vi "Remote Panels Handler.vi"(8 "error in (no error)":errorcluster, 10 "Limit  connections":i32=1 min=1, 11 "VI in":refnum<vi>) -> (0 "error out":errorcluster, 3 "VI out":refnum<vi>)   [LabVIEW 2018]
uses:
  Remote Panels Globals.vi
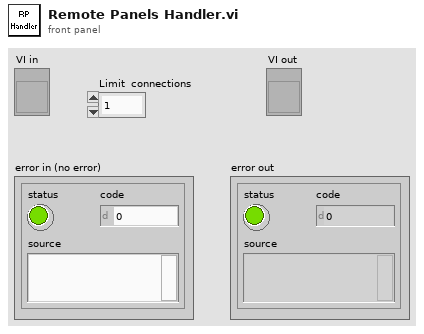
[diagram p1: front panel]
types:
  T1 = enum32{"Bad", "Idle", "Run top level", "Running"}
  T2 = typedef "LVRemotePanelConnectionsTypeDef.ctl" = cluster{"VI Name":string, "Remote":string, "UserName":string, "Port":i32, "Status":enum32{"Viewing", "Waiting For Control", "Controlling"}, "Create Time":timestamp, "Status Time":timestamp, "Control End Time":timestamp}[]
  T3 = cluster{"VI Name":string, "Remote":string, "UserName":string, "Port":i32, "Status":enum32{"Viewing", "Waiting For Control", "Controlling"}, "Create Time":timestamp, "Status Time":timestamp, "Control End Time":timestamp}
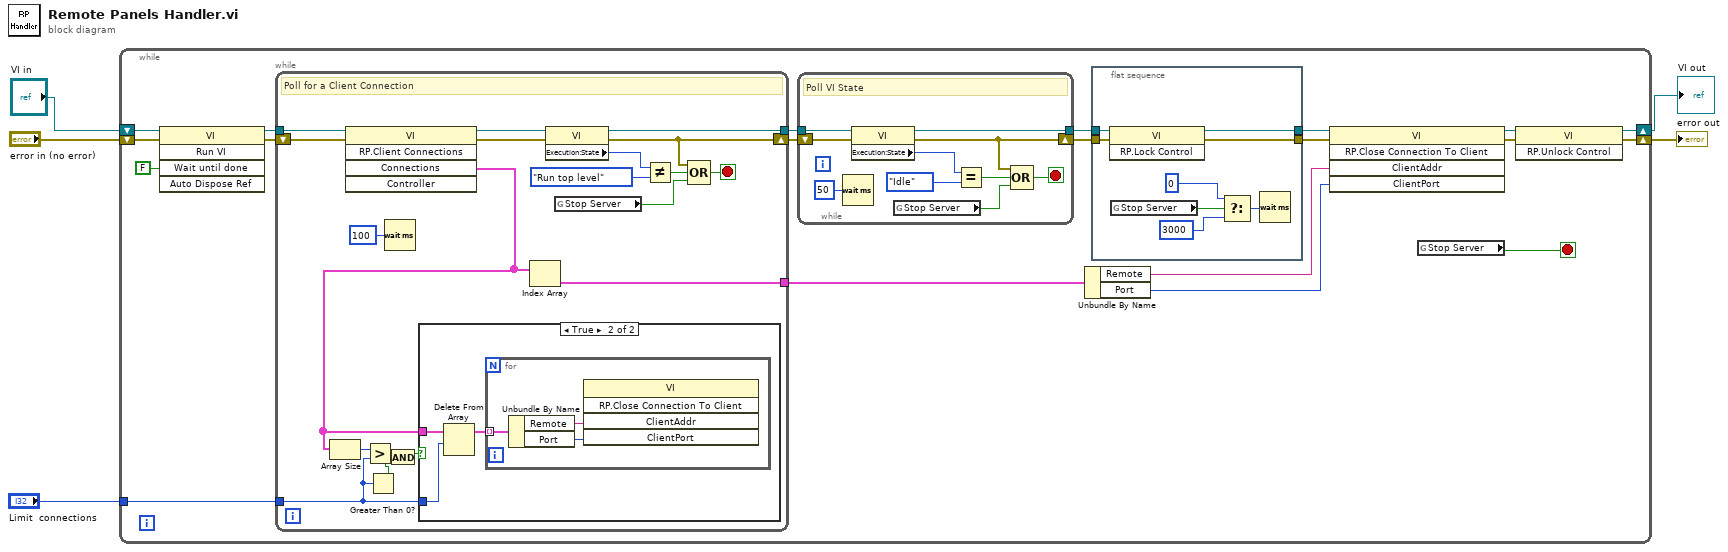
[diagram p0: block diagram]
diagram:
  n1 = while {
    shift-right: [w22] -> w3
    shift-left: "error in (no error)" -> [w8]
    shift-right: [w23] -> w2
    shift-left: "VI in" -> [w10]
    tunnel: "Limit  connections" -> [w6]
    stop <- w12 stop-if-true
    n2 = invoke class="VI" method="Run VI"(reference=w10, error in=w8, "Wait until done"=FALSE ("Wait Until Done")) -> (reference out=w9:refnum<vi>, error out=w7:errorcluster)  [unwired: 2 in, 3 out]
    n3 = while {
      tunnel: w9 -> [w51]
      tunnel: [w54] -> w20
      shift-right: [w53] -> w21
      shift-left: w7 -> [w60]
      tunnel: [w52] -> w13
      tunnel: w6 -> [w46]
      stop <- w61 stop-if-true
      # "Poll for a Client Connection"
      n4 = invoke class="VI" method="RP.Client Connections"(reference=w51, error in=w60) -> (reference out=w55:refnum<vi>, error out=w57:errorcluster, "Connections"=w47:T2)  [unwired: 3 in, 2 out]
      n5 = Array Size(array=w47) -> (size(s)=w48:i32)
      n6 = Greater?(x=w48, y=w46) -> (0:w49:bool)
      n7 = Greater Than 0?(x=w46) -> (x > 0?=w44:bool)
      n8 = Wait (ms)(milliseconds to wait=u32 100) -> ()  [unwired: 1 out]
      n9 = And(x=w49, y=w44) -> (x .and. y?=w45:bool)
      n10 = case shown="True" w45 {
        tunnel: w47 -> [_ w65]
        tunnel: w46 -> [_ w63]
        frame False {
        }
        frame True {
          n11 = Delete From Array(array=w65, length=w63) -> (array with subset deleted=w64:T2)  [unwired: 1 in, 1 out]
          n12 = for {
            tunnel: w64 -> [w68] mode=indexing
            n13 = Unbundle By Name(w68) -> ("Remote"=w67:string, "Port"=w66:i32)
            n14 = invoke class="VI" method="RP.Close Connection To Client"("ClientAddr"=w67, "ClientPort"=w66) -> ()  [unwired: 3 in, 5 out]
          }
        }
      }
      n15 = Index Array(array=w47) -> (element=w52:T3)  [unwired: 1 in]
      n16 = property class="VI"(reference=w55, error in=w57) -> (reference out=w54:refnum<vi>, error out=w53:errorcluster, "Execution:State"=w59:T1)
      n17 = global read "Remote Panels Globals.vi" "Stop Server"() -> (w50:bool)
      n18 = Not Equal?(x=w59, y=T1."Run top level" ("Execution:State")) -> (x != y?=w56:bool)
      n19 = Compound Arithmetic op=OR(w53, w56, w50) -> (w61:bool)
    }
    n20 = while {
      tunnel: w20 -> [w41]
      tunnel: [w36] -> w16
      shift-right: [w35] -> w19
      shift-left: w21 -> [w43]
      stop <- w38 stop-if-true
      # "Poll VI State"
      n21 = Wait (ms)(milliseconds to wait=u32 50) -> ()  [unwired: 1 out]
      n22 = property class="VI"(reference=w41, error in=w43) -> (reference out=w36:refnum<vi>, error out=w35:errorcluster, "Execution:State"=w40:T1)
      n23 = global read "Remote Panels Globals.vi" "Stop Server"() -> (w34:bool)
      n24 = Equal?(x=w40, y=T1."Idle" ("Execution:State")) -> (x = y?=w37:bool)
      n25 = Compound Arithmetic op=OR(w35, w37, w34) -> (w38:bool)
    }
    n26 = Unbundle By Name(w13) -> ("Remote"=w15:string, "Port"=w14:i32)
    n27 = flat-sequence {
      tunnel: w19 -> [w33]
      tunnel: [w32] -> w18
      tunnel: [w31] -> w17
      tunnel: w16 -> [w26]
      frame #0 {
        n28 = invoke class="VI" method="RP.Lock Control"(reference=w26, error in=w33) -> (reference out=w31:refnum<vi>, error out=w32:errorcluster)  [unwired: 1 in, 1 out]
        n29 = global read "Remote Panels Globals.vi" "Stop Server"() -> (w30:bool)
        n30 = Select(t=u32 0 ("milliseconds to wait"), s=w30, f=u32 3000 ("milliseconds to wait")) -> (s? t:f=w27:u32)
        n31 = Wait (ms)(milliseconds to wait=w27) -> ()  [unwired: 1 out]
      }
    }
    n32 = invoke class="VI" method="RP.Close Connection To Client"(reference=w17, error in=w18, "ClientAddr"=w15, "ClientPort"=w14) -> (reference out=w24:refnum<vi>, error out=w25:errorcluster)  [unwired: 1 in, 3 out]
    n33 = global read "Remote Panels Globals.vi" "Stop Server"() -> (w12:bool)
    n34 = invoke class="VI" method="RP.Unlock Control"(reference=w24, error in=w25) -> (reference out=w23:refnum<vi>, error out=w22:errorcluster)  [unwired: 1 in, 1 out]
  }
  "error out" <- w3
  "VI out" <- w2
